vi "Export NI-SWITCH Custom Device.vi"(8 "error in":errorcluster, 9 "operation":T1(ring)=enum."replace or create with confirmation", 10 "datalog path (use dialog)":path, 11 "ni-switch custom device in":T2 format="%.0x") -> (0 "error out":errorcluster, 3 "ni-switch custom device out":T2 format="%.0x")   [LabVIEW 2017, in "NI-SWITCH Scripting.lvlib"]
doc: "Saves the configuration for the SLSC Switch custom device as a datalog file. Import the datalog file by using <b>Import SLSC Switch Custom Device.vi</b>."
uses:
  NI-SWITCH Scripting.lvlib
  <vilib>/NI Veristand/Custom Device API/Custom Device Item Ref.ctl
  <vilib>/NI/NI VeriStand Custom Device Import and Export Tool/ImportExport.lvlib
  <vilib>/NI VeriStand/Custom Device API/Custom Device API.lvlib
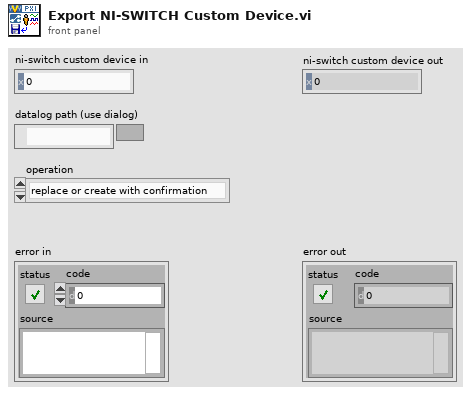
[diagram p1: front panel]
types:
  T1 = enum16{"open", "replace", "create", "open or create", "replace or create", "replace or create with confirmation"}
  T2 = typedef "Custom Device API.lvlib/Custom Device Item Ref.ctl" = u64
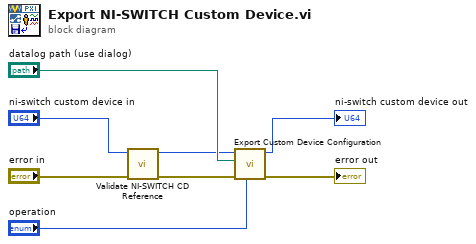
[diagram p0: block diagram]
diagram:
  n1 = call "Validate NI-SWITCH CD Reference.vi"("error in"="error in", "ni-switch custom device in"="ni-switch custom device in") -> ("error out"=w3:errorcluster, "ni-switch custom device out"=w2:T2)  [unwired: 8 in]
  n2 = call <vilib>:"Export Custom Device Configuration.vi"("operation"="operation", "error in (no error)"=w3, "Path"="datalog path (use dialog)", "ID"=w2) -> ("error out"=→"error out":errorcluster, "ID out"=→"ni-switch custom device out":u64)  [unwired: 6 in]
